vi "Change_V_Range.vi"() -> ()   [LabVIEW 2020]
panel:
  in  "Keysense":string
  in  "VRange_Value":string="VRange"
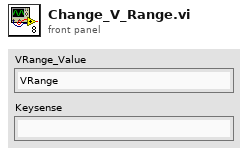
[diagram p1: front panel]
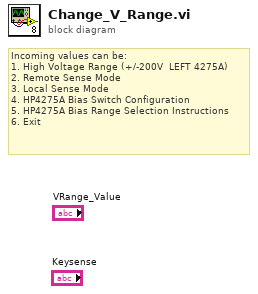
[diagram p0: block diagram]
diagram:
  # "Incoming values can be:\n1. High Voltage Range (+/-200V  LEFT 4275A)\n2. Remote Sense Mode\n3. Local Sense Mode\n4. HP4275A Bias Switch Configuration\n5. HP4275A Bias Range Selection Instructions\n6. Exit"
